vi "EMD8216 IP change.vi"(9 "IP":u8[](array[numeric]), 11 "CardID":u32) -> (3 "error_code":u32)   [LabVIEW 2009, in "EMD8216_64.lvlib"]
doc: "EMD8216Status EMD8216_IP_change(u32 CardID,u8 IP[4]);"
uses:
  EMD8216_64.lvlib
  <userlib>/EMD8216_64/EMD8216_64.dll
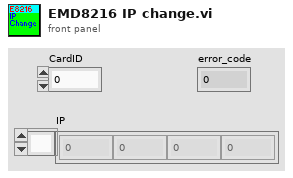
[diagram p1: front panel]
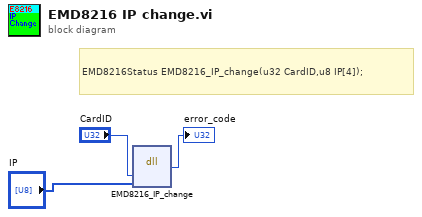
[diagram p0: block diagram]
diagram:
  # "EMD8216Status EMD8216_IP_change(u32 CardID,u8 IP[4]);"
  n1 = dll-call lib="C:/Program Files/National Instruments/LabVIEW 2017/user.lib/EMD8216_64/EMD8216_64.*" fn="EMD8216_IP_change"("CardID"="CardID", "IP"="IP") -> ("return type"=→"error_code":u32)  [unwired: 5 in, 2 out]
